vi "update_id_ajuste_previo.vi"(8 "error in (no error)":errorcluster, 11 "Base de Datos in":refnum<class "Base de Datos.lvclass">) -> (0 "error out":errorcluster, 2 "last_id_ajuste_previo":i32, 3 "Base de Datos out":refnum<class "Base de Datos.lvclass">)   [LabVIEW 2019, in "Base de Datos.lvclass"]
uses:
  Base de Datos.lvclass
  Globals/globales.vi
  SQLiteConnector/SQLiteConnection.lvclass
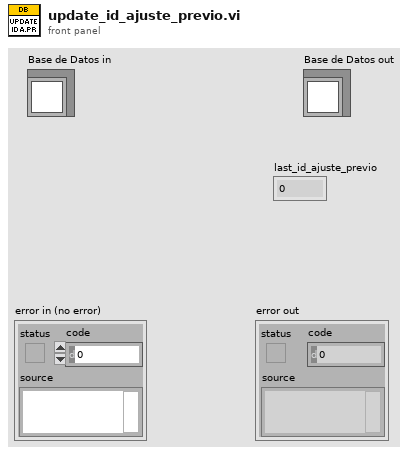
[diagram p1: front panel]
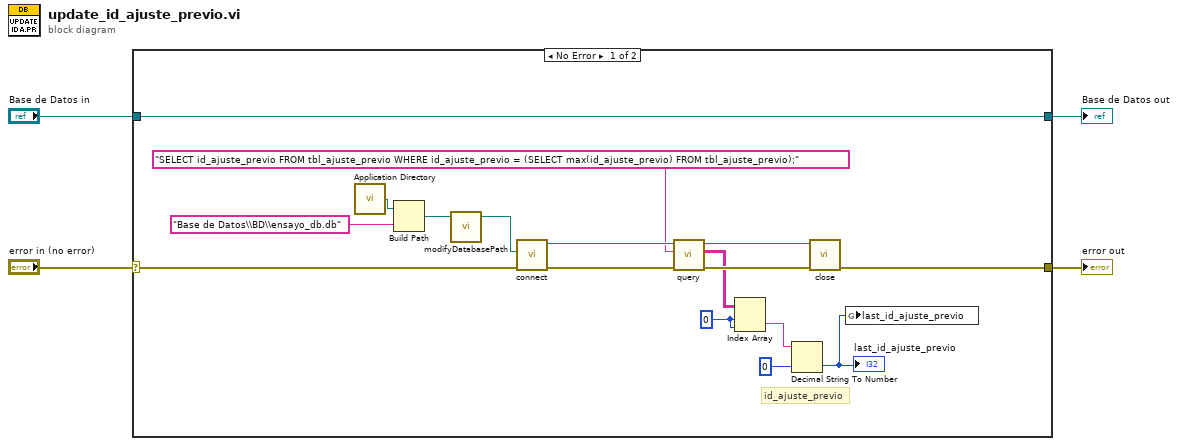
[diagram p0: block diagram]
diagram:
  n1 = case shown="No Error" "error in (no error)" {
    selector: "error in (no error)" -> [w5 w22]
    tunnel: [w15 w22] -> w4
    tunnel: [w6 w23] -> w3
    tunnel: "Base de Datos in" -> [w6 w23]
    frame No Error {
      w11 = 0 ("index (row)")
      # "id_ajuste_previo"
      n2 = call <vilib>:"Application Directory.vi"() -> ("Application Directory"=w21:path)
      n3 = Build Path(base path=w21, name or relative path="Base de Datos\\BD\\ensayo_db.db" ("BD")) -> (appended path=w20:path)
      n4 = call "modifyDatabasePath.vi"("Database Path In"=w20) -> ("Database Path Out"=w19:path)  [unwired: 4 in]
      n5 = call "connect.vi"("error in (no error)"=w5, "Database Path"=w19) -> ("error out"=w16:errorcluster, "object out"=w17:refnum<class "SQLiteConnection.lvclass">)  [unwired: 8 in]
      n6 = call "query.vi"("error in (no error)"=w16, "SQL Statement"="SELECT id_ajuste_previo FROM tbl_ajuste_previo WHERE id_ajuste_previo = (SELECT max(id_ajuste_previo) FROM tbl_ajuste_previo);" ("format string"), "object in"=w17) -> ("error out"=w14:errorcluster, "result"=w12:string[][], "object out"=w13:refnum<class "SQLiteConnection.lvclass">)  [unwired: 5 in, 1 out]
      n7 = Index Array(array=w12, index (row)=w11, index (col)=w11) -> (element=w10:string)
      n8 = Decimal String To Number(string=w10, default (0L)=0) -> (number=w8:i32)  [unwired: 1 in, 1 out]
      "last_id_ajuste_previo" <- w8
      n9 = call-dynamic "close.vi"("error in (no error)"=w14, "object in"=w13) -> ("error out"=w15:errorcluster)  [unwired: 8 in, 1 out]
      n10 = global write "globales.vi" "last_id_ajuste_previo"(w8) -> ()
    }
    frame Error {
    }
  }
  "error out" <- w4
  "Base de Datos out" <- w3
